vi "TDMS.GetIteration.vi"(8 "error in (no error)":errorcluster, 11 "Data":path) -> (0 "error out":errorcluster, 2 "Iteration":i32, 3 "tdms file out":refnum<k34>)   [LabVIEW 2015, in "NIAnalysis.lvlib"]
uses:
  NIAnalysis.lvlib
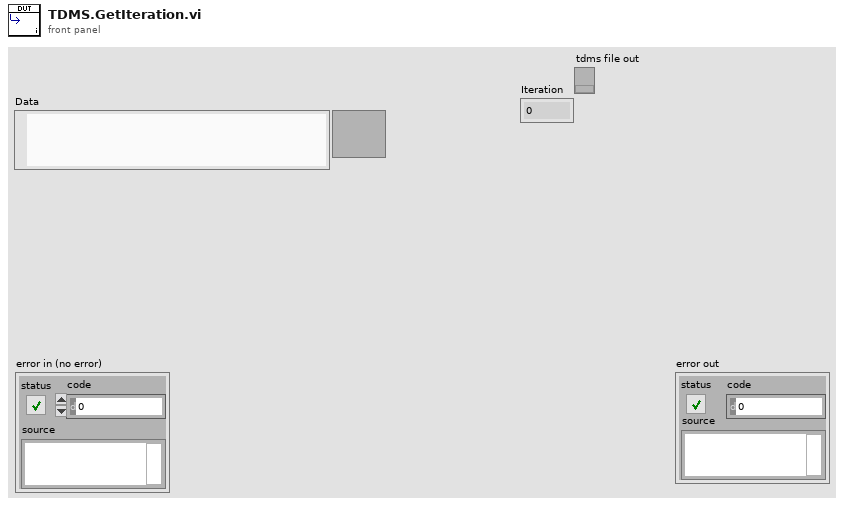
[diagram p1: front panel]
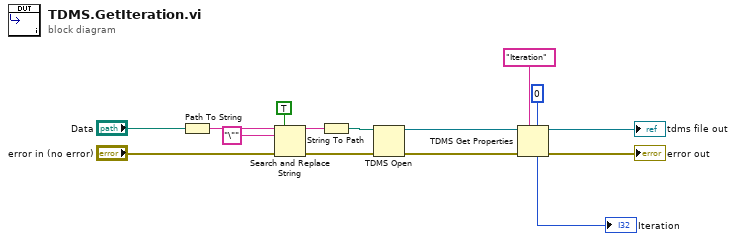
[diagram p0: block diagram]
diagram:
  n1 = Path To String(path="Data") -> (string=w14:string)
  n2 = Search and Replace String(replace all?=TRUE ("replace all? (F)"), input string=w14, search string="\"", error in="error in (no error)") -> (result string=w15:string, error out=w9:errorcluster)  [unwired: 4 in, 2 out]
  n3 = String To Path(string=w15) -> (path=w10:path)
  n4 = TDMS Open(8:w9, 11:w10) -> (0:w7:errorcluster, 3:w8:refnum<k34>)  [unwired: 5 in]
  n5 = TDMS Get Properties(5:0 ("Iteration"), 7:"Iteration" ("Iteration.Property"), 8:w7, 11:w8) -> (0:→"error out":errorcluster, 3:→"tdms file out":refnum<k34>, 4:→"Iteration":i32)  [unwired: 2 in, 3 out]
